vi "simple example.vi"() -> ()   [LabVIEW 2020]
uses:
  reqwest/header.ctl
  reqwest/reqwest.lvclass
panel:
  out "Duration":dbl
  out "error out":errorcluster
  out "response":string
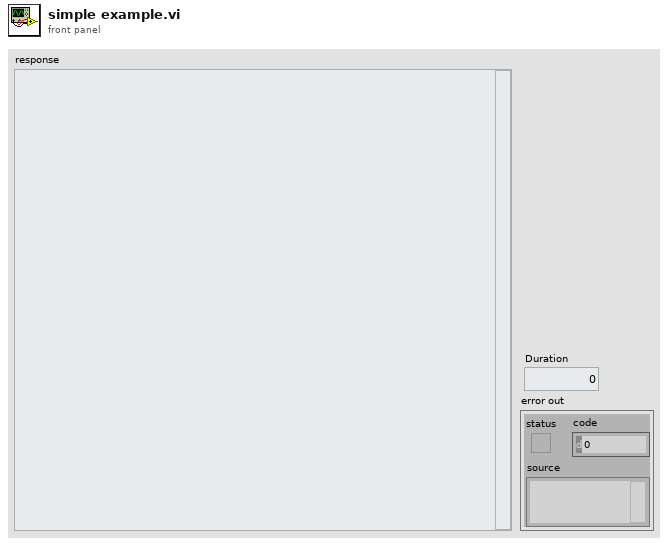
[diagram p1: front panel]
types:
  T1 = typedef "reqwest.lvclass/header.ctl" = cluster{"header":string, "value":string}
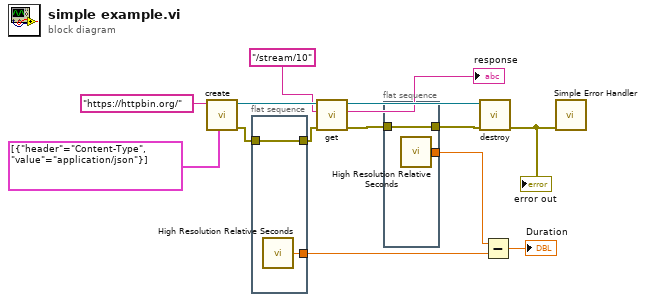
[diagram p0: block diagram]
diagram:
  n1 = call "create.vi"("Default Headers ([JSON])"=T1[] [{"header"="Content-Type", "value"="application/json"}], "Base URL"="https://httpbin.org/") -> ("error out"=w8:errorcluster, "reqwest"=w13:refnum<class "reqwest.lvclass">)  [unwired: 8 in]
  n2 = flat-sequence {
    tunnel: w8 -> [w16]
    tunnel: [w16] -> w7
    tunnel: [w15] -> w3
    frame #0 {
      n3 = call <vilib>:"High Resolution Relative Seconds.vi"() -> ("relative seconds"=w15:dbl)
    }
  }
  n4 = call "get.vi"("error in (no error)"=w7, "path"="/stream/10", "reqwest in"=w13) -> ("error out"=w6:errorcluster, "response"=→"response":string, "reqwest out"=w12:refnum<class "reqwest.lvclass">)  [unwired: 6 in]
  n5 = flat-sequence {
    tunnel: w6 -> [w18]
    tunnel: [w18] -> w5
    tunnel: [w17] -> w4
    frame #0 {
      n6 = call <vilib>:"High Resolution Relative Seconds.vi"() -> ("relative seconds"=w17:dbl)
    }
  }
  n7 = call "destroy.vi"("error in (no error)"=w5, "reqwest"=w12) -> ("error out"=w9:errorcluster)  [unwired: 9 in]
  "error out" <- w9
  n8 = Subtract(x=w4, y=w3) -> (x-y=→"Duration":dbl)
  n9 = call <vilib>:"Simple Error Handler.vi"("error in (no error)"=w9) -> ()  [unwired: 4 in, 5 out]
